vi "Write text.vi"(8 "error in (no error)":errorcluster, 10 "text":string, 11 "TextDecoration in":refnum<class "TextDecoration.lvclass">) -> (0 "error out":errorcluster, 3 "TextDecoration out":refnum<class "TextDecoration.lvclass">)   [LabVIEW 2023, in "TLC_Scripto.lvlib" / "TextDecoration.lvclass"]
uses:
  TextDecoration.lvclass
  Read textDecorationRef.vi
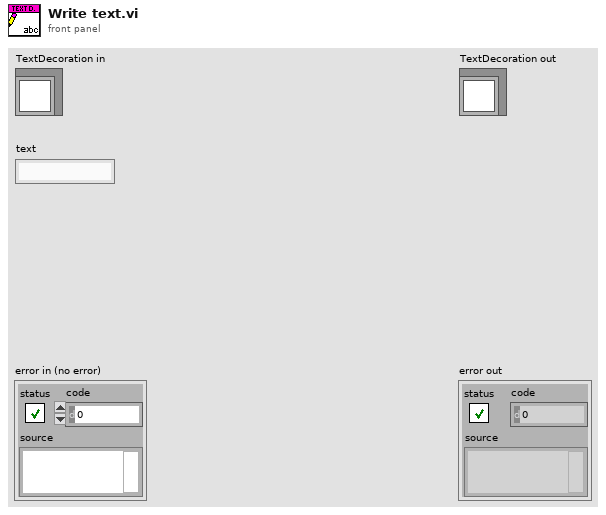
[diagram p1: front panel]
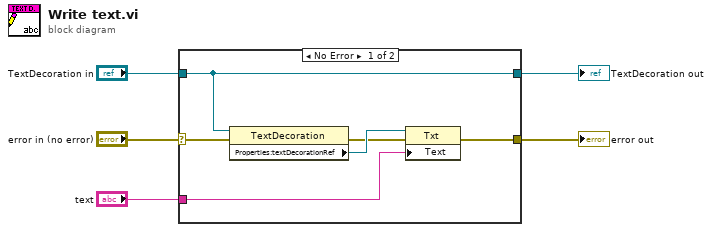
[diagram p0: block diagram]
diagram:
  n1 = case shown="No Error" "error in (no error)" {
    selector: "error in (no error)" -> [w9 w12]
    tunnel: [w8 w12] -> w4
    tunnel: [w6 w13] -> w2
    tunnel: "TextDecoration in" -> [w6 w13]
    tunnel: "text" -> [w7 _]
    frame No Error {
      n2 = property class="TextDecoration"(reference=w6, error in=w9) -> (error out=w10:errorcluster, "Properties:textDecorationRef"=w11:refnum<vi>)  [unwired: 1 out]
      n3 = property class="Txt"(reference=w11, error in=w10, "Text"=w7) -> (error out=w8:errorcluster)  [unwired: 1 out]
    }
    frame Error {
    }
  }
  "error out" <- w4
  "TextDecoration out" <- w2
